vi "IntakeUntilBall-C.vi"(11 "Params":string[][](array[string])) -> ()   [LabVIEW 2018]
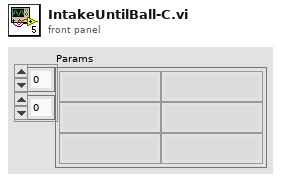
[diagram p1: front panel]
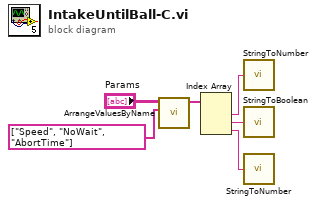
[diagram p0: block diagram]
diagram:
  n1 = call "ArrangeValuesByName.vi"("Names"=string[] ["Speed", "NoWait", "AbortTime"], "Names/Values in"="Params") -> ("Values Out"=w4:string[])  [unwired: 9 in]
  n2 = Index Array(array=w4) -> (element #1=w3:string, element #2=w2:string, element #3=w1:string)  [unwired: 3 in]
  n3 = call "StringToNumber.vi"("String"=w3) -> ()  [unwired: 1 out]
  n4 = call "StringToBoolean.vi"("String"=w2) -> ()  [unwired: 1 out]
  n5 = call "StringToNumber.vi"("String"=w1) -> ()  [unwired: 1 out]
